vi "actualiza botones.vi"(10 "Controls[]":refnum<vi>[](array[refnum]), 11 "Array":T1(array[cluster])) -> ()   [LabVIEW 2020, in "Productos.lvlib"]
uses:
  Productos.lvlib
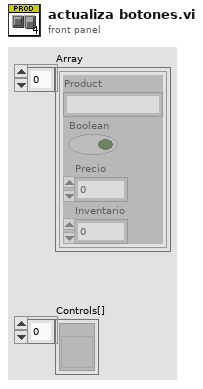
[diagram p1: front panel]
types:
  T1 = cluster{"Product":string, "Boolean":bool, "Precio":dbl, "Inventario":dbl}[]
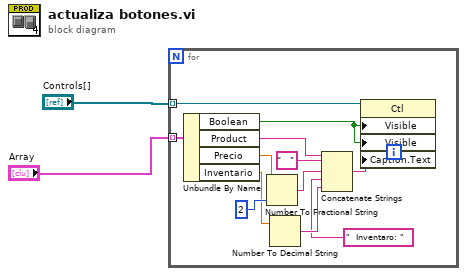
[diagram p0: block diagram]
diagram:
  n1 = for {
    tunnel: "Controls[]" -> [w14] mode=indexing
    tunnel: "Array" -> [w13] mode=indexing
    n2 = Unbundle By Name(w13) -> ("Boolean"=w10:bool, "Product"=w9:string, "Precio"=w12:dbl, "Inventario"=w5:dbl)
    n3 = Number To Fractional String(number=w12, precision (6)=i16 2) -> (F-format string=w6:string)  [unwired: 2 in]
    n4 = Number To Decimal String(number=w5) -> (decimal integer string=w4:string)  [unwired: 1 in]
    n5 = Concatenate Strings(w9, "   " ("string"), w6, "  Inventaro: " ("string"), w4) -> (w8:string)
    n6 = property class="Ctl"(reference=w14, "Visible"=w10, "Visible"=w10, "Caption.Text"=w8) -> ()  [unwired: 1 in, 2 out]
  }
